vi "Main2.vi"() -> ()   [LabVIEW 2014]
uses:
  Enum State Typedef.ctl
  <vilib>/Utility/error.llb/DialogType.ctl
  <vilib>/_DAQmxBase/Internals/DAQmxBase Create Channel (AI-Voltage-Basic).vi
  <vilib>/_DAQmxBase/Internals/DAQmxBase Timing (Sample Clock).vi
  <vilib>/_DAQmxBase/Internals/DAQmxBase Read (Analog 2D DBL NChan NSamp).vi
  <vilib>/Utility/file.llb/Write To Spreadsheet File (DBL).vi
panel:
  out "State":T1
  in  "Clear Display":bool
  in  "Preview Button":bool
  out "size(s)":i32
  in  "pH":dbl
  in  "Conductivity (mS)":dbl
  out "Iterations Recorded":i32
  in  "Recording Time (seconds)":dbl
  in  "Sample Rate":i32=1000
  in  "physical channels":tag
  in  "Stop Button":bool
  out "Waveform Chart":waveform(dbl)(graph)
  in  "High Pass Filter":enum16{"500", "1k", "5k", "10k", "20k"}(ring)
  in  "Low Pass Filter":enum16{"0.1", "1.0", "10", "100", "300"}(ring)
  in  "Gain":enum16{"x100", "x1000", "x10k"}(ring)
  in  "Notch Filter":bool
  in  "Amplifier Model":u16(ring) items=["Select a Model", "AM 1700", "BMA 200"]
  in  "AC/DC Switch":bool
  in  "Temperature (deg C)":dbl
  in  "User Comments":string
  out "Start Time hr/min":string
  out "Date mm/dd/yy":string
  in  "Species":string
  in  "Exit Button":bool
  in  "Record Button":bool
  # "MSU EFISH Lab Single Channel Electronic Pulse Recorder"
  # "Must enter numbers into here before you run"
  # "Blue for On\nOrange for Off"
  # "DC"
  # "AC"
  # "Blue for AC and Orange for DC"
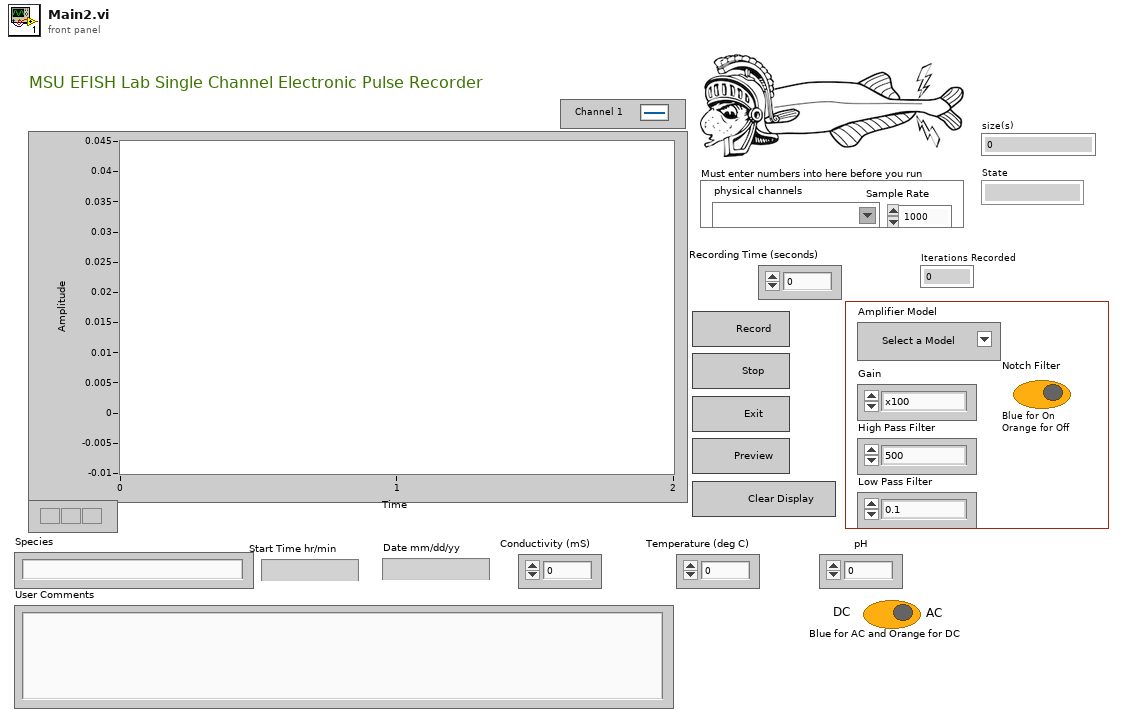
[diagram p1: front panel]
types:
  T1 = typedef "Enum State Typedef.ctl" = enum16{"", "Prepreview Handling", "Clear Display", "Preview Data", "Stop", "Exit", "Record", "Create File"}
  T2 = typedef "DialogType.ctl" = u16
  T3 = cluster{"High Pass Filter":enum16{"500", "1k", "5k", "10k", "20k"}, "Gain":enum16{"x100", "x1000", "x10k"}, "Low Pass Filter":enum16{"0.1", "1.0", "10", "100", "300"}, "Amplifier Model":u16, "Notch Filter":bool, "AC/DC Switch":bool, "Temperature (deg C)":dbl, "Conductivity (mS)":dbl, "pH":dbl, "User Comments":string, "Species":string}
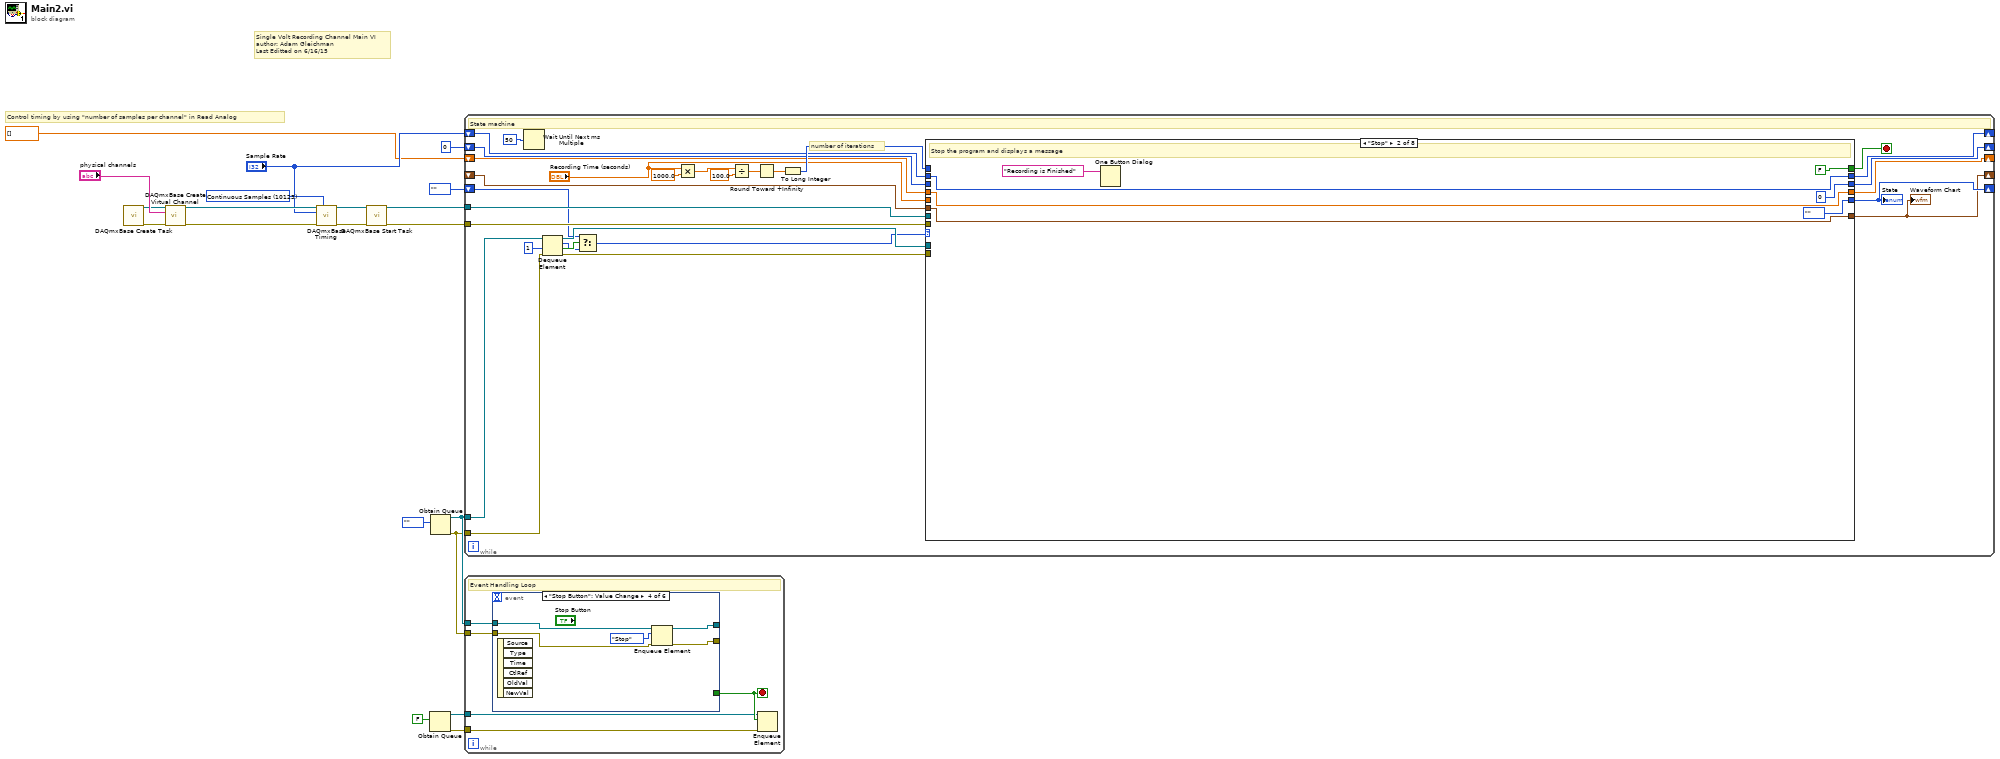
[diagram p0: block diagram]
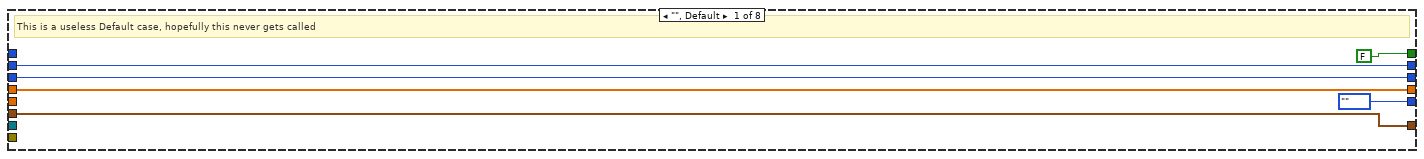
[diagram p2: hidden frame]
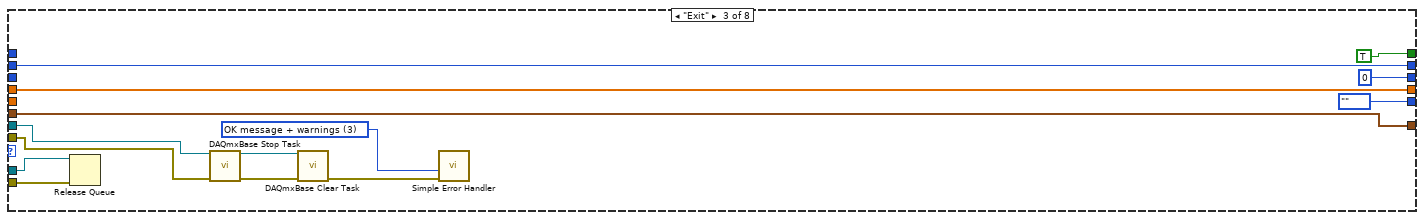
[diagram p3: hidden frame]
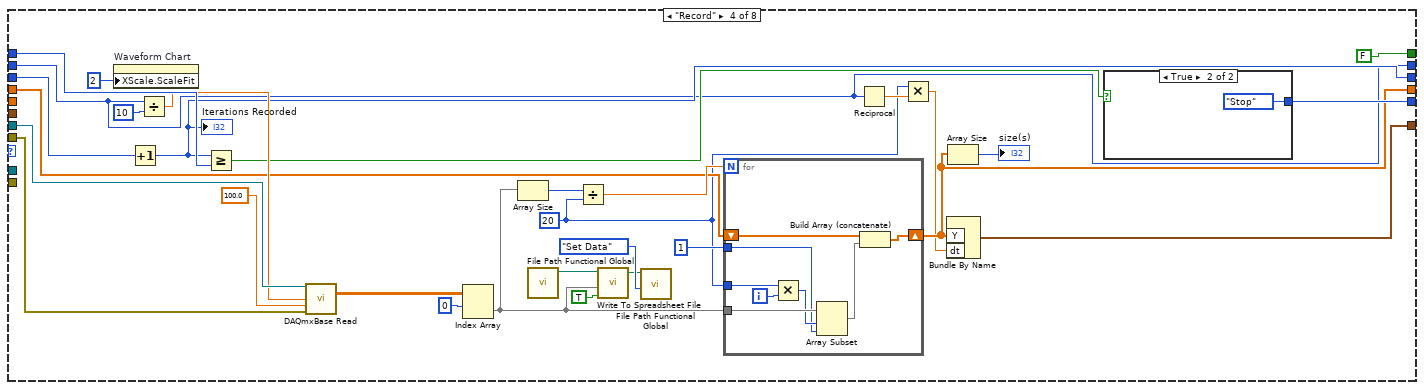
[diagram p4: hidden frame]
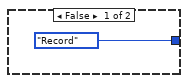
[diagram p5: hidden frame]
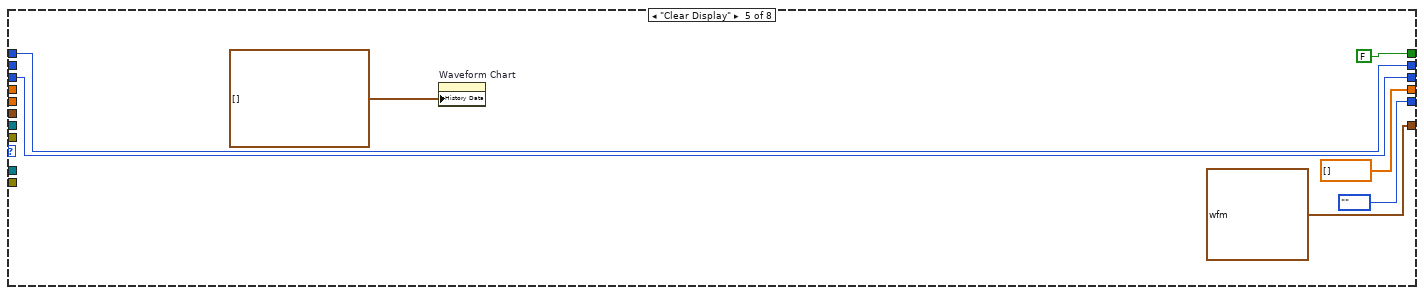
[diagram p6: hidden frame]
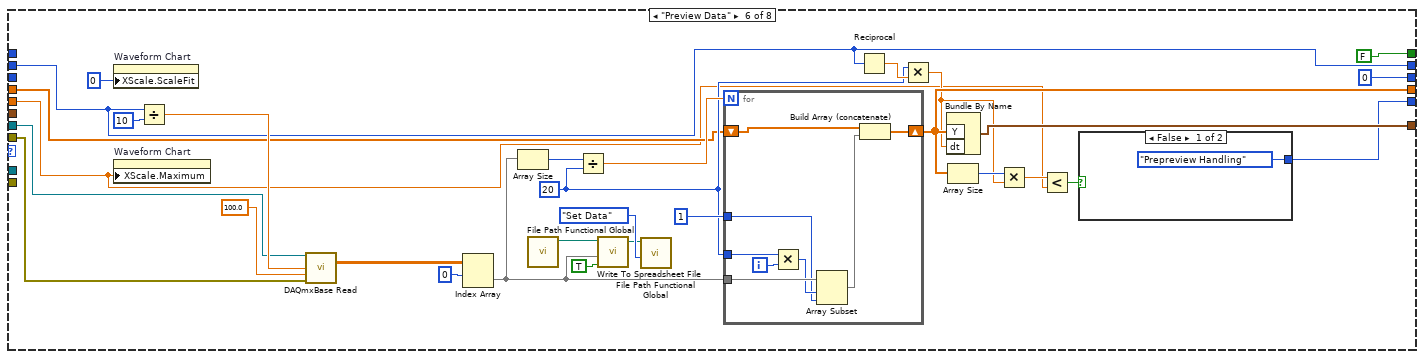
[diagram p7: hidden frame]
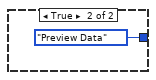
[diagram p8: hidden frame]
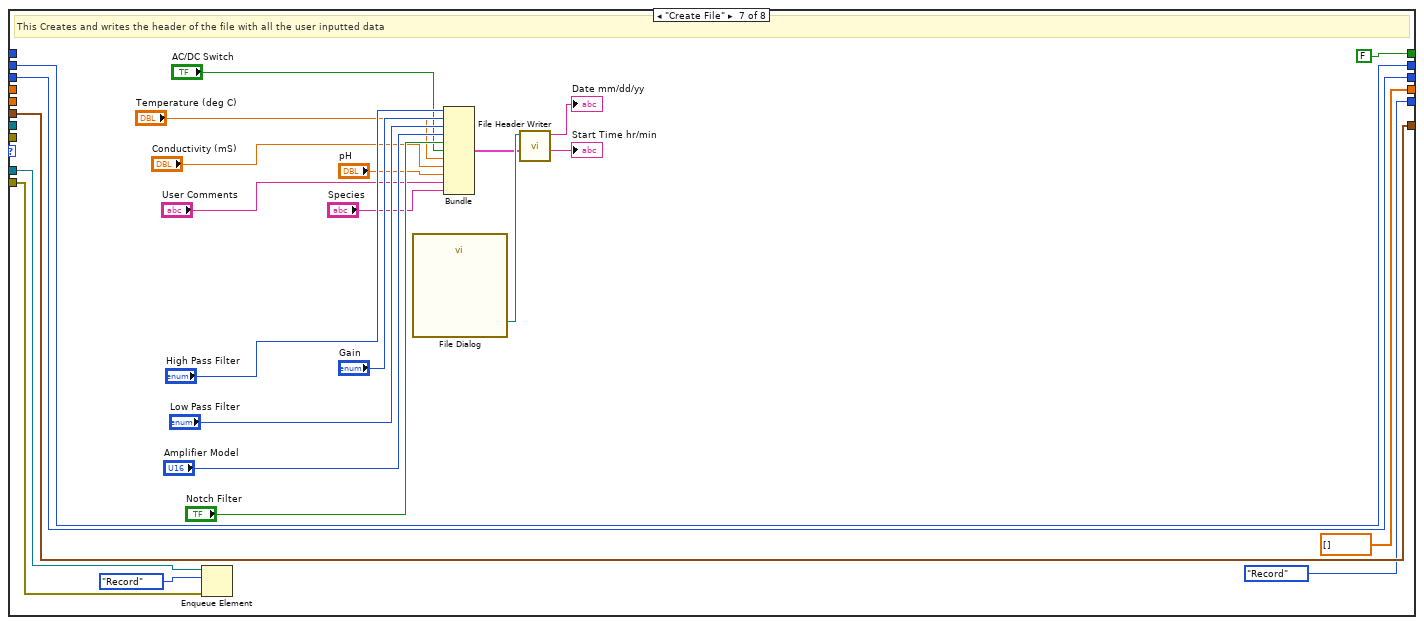
[diagram p9: hidden frame]
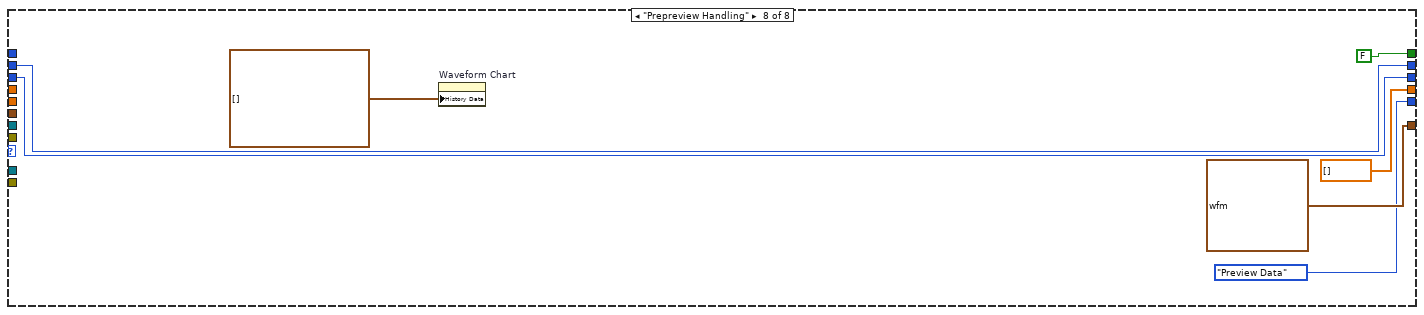
[diagram p10: hidden frame]
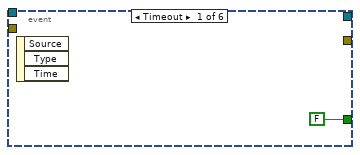
[diagram p11: hidden frame]
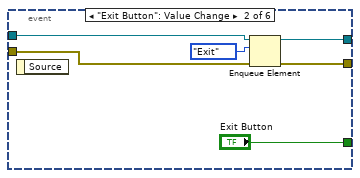
[diagram p12: hidden frame]
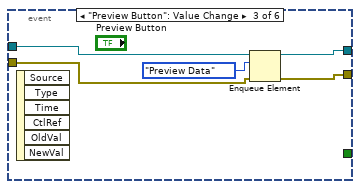
[diagram p13: hidden frame]
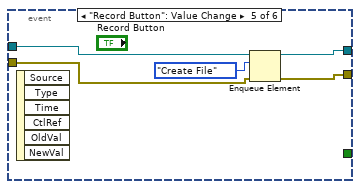
[diagram p14: hidden frame]
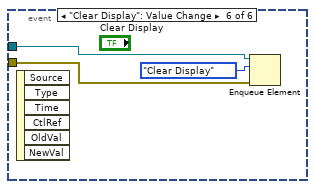
[diagram p15: hidden frame]
diagram:
  w12 = 10123 items=["Finite Samples"=10178, "Continuous Samples"=10123, "Hardware Timed Single Point"=12522] ("sample mode")
  # "Single Volt Recording Channel Main VI\nauthor: Adam Gleichman\nLast Editted on 6/16/15"
  # "Control timing by using \"number of samples per channel\" in Read Analog"
  n1 = call <vilib>:"DAQmxBase Create Task.vi"() -> ("task out"=w16:refnum<k21>, "error out"=w15:errorcluster)  [unwired: 14 in]
  n2 = call-poly <vilib>:"DAQmxBase Create Virtual Channel.vi"("task in"=w16, "physical channels"="physical channels", "error in"=w15) -> ("task out"=w14:refnum<k21>, "error out"=w13:errorcluster)  [unwired: 11 in]
  n3 = call-poly <vilib>:"DAQmxBase Timing.vi"("task/channels in"=w14, "sample mode"=w12, "rate"="Sample Rate", "error in"=w13) -> ("task out"=w11:refnum<k21>, "error out"=w10:errorcluster)  [unwired: 10 in]
  n4 = call <vilib>:"DAQmxBase Start Task.vi"("task/channels in"=w11, "error in"=w10) -> ("task out"=w8:refnum<k21>, "error out"=w9:errorcluster)  [unwired: 12 in]
  n5 = Obtain Queue(element data type=FALSE) -> (queue out=w2:refnum<queue>, error out=w1:errorcluster)  [unwired: 4 in, 1 out]
  n6 = Obtain Queue(element data type=Enum_State_Typedef."" ("State")) -> (queue out=w19:refnum<queue>, error out=w18:errorcluster)  [unwired: 4 in, 1 out]
  n7 = while {
    tunnel: w19 -> [w49]
    tunnel: w18 -> [w48]
    tunnel: w9 -> [w43]
    tunnel: w8 -> [w44]
    shift-right: [w35] -> _
    shift-left: 0 -> [w36]
    shift-right: [w30] -> _
    shift-left: Enum_State_Typedef."" ("State") -> [w32]
    shift-right: [w28] -> _
    shift-left: "Sample Rate" -> [w29]
    shift-right: [w22] -> _
    shift-left: dbl[] [] -> [w25]
    shift-right: [w24] -> _
    shift-left: _ -> [w23]
    stop <- w47 stop-if-true
    # "number of iterations"
    # "State machine"
    n8 = Wait Until Next ms Multiple(millisecond multiple=u32 50) -> ()  [unwired: 1 out]
    n9 = Dequeue Element(queue=w49, timeout in ms (-1)=1, error in (no error)=w48) -> (queue out=w46:refnum<queue>, element=w33:T1, timed out?=w34:bool, error out=w45:errorcluster)
    n10 = Select(t=w32, s=w34, f=w33) -> (s? t:f=w31:T1)
    n11 = Multiply(x="Recording Time (seconds)", y=1000.0) -> (x*y=w41:dbl)
    n12 = Divide(x=w41, y=100.0) -> (x/y=w39:dbl)
    n13 = Round Toward +Infinity(x=w39) -> (ceil(x): smallest int >= x=w38:dbl)
    n14 = To Long Integer(number=w38) -> (32bit integer=w37:i32)
    n15 = case shown="\"Stop\"" w31 {
      tunnel: [FALSE FALSE TRUE FALSE FALSE FALSE FALSE FALSE] -> w47
      tunnel: w46 -> [_ _ w69 _ _ _ w187 _]
      tunnel: w45 -> [_ _ w68 _ _ _ w186 _]
      tunnel: w44 -> [_ _ w73 w105 _ w135 _ _]
      tunnel: w43 -> [_ _ w72 w104 _ w134 _ _]
      tunnel: w29 -> [w52 w59 w65 w81 _ w130 w183 w189]
      tunnel: w37 -> [_ _ _ w97 w120 _ _ _]
      tunnel: w36 -> [w54 _ _ w98 w123 _ w184 w190]
      tunnel: [w54 0 0 w92 w123 0 w184 w190] -> w35
      tunnel: [Enum_State_Typedef."" ("State") Enum_State_Typedef."" ("State") Enum_State_Typedef."" ("State") w94 Enum_State_Typedef."" ("State") w132 Enum_State_Typedef."Record" ("State") Enum_State_Typedef."Preview Data" ("State")] -> w30
      tunnel: [w52 w59 w65 w81 w120 w130 w183 w189] -> w28
      tunnel: [w51 w57 w64 w85 dbl[] [] w131 dbl[] [] dbl[] []] -> w22
      tunnel: w25 -> [w51 w57 w64 w84 _ w136 _ _]
      tunnel: [w50 w56 w63 w83 waveform(dbl) {"t0"=timestamp(0 s since 1904-01-01), "dt"=1.0, "Y"=[]} w133 w171 waveform(dbl) {"t0"=timestamp(0 s since 1904-01-01), "dt"=1.0, "Y"=[]}] -> w24
      tunnel: w23 -> [w50 w56 w63 _ _ _ w171 _]
      tunnel: "Recording Time (seconds)" -> [_ _ _ _ _ w125 _ _]
      frame "", Default {
        # "This is a useless Default case, hopefully this never gets called"
      }
      frame "Stop" {
        # "Stop the program and displays a message"
        n16 = One Button Dialog(message="Recording is Finished") -> ()  [unwired: 1 in, 1 out]
      }
      frame "Exit" {
        w70 = T2 3 items=["no dialog", "OK message", "continue or stop message", "OK message + warnings", "continue/stop + warnings"] ("type of dialog (OK msg:1)")
        n17 = Release Queue(queue=w69, error in (no error)=w68) -> ()  [unwired: 1 in, 3 out]
        n18 = call <vilib>:"DAQmxBase Stop Task.vi"("task/channels in"=w73, "error in"=w72) -> ("task out"=w75:refnum<k21>, "error out"=w74:errorcluster)  [unwired: 12 in]
        n19 = call <vilib>:"DAQmxBase Clear Task.vi"("task in"=w75, "error in"=w74) -> ("error out"=w71:errorcluster)  [unwired: 13 in]
        n20 = call <vilib>:"Simple Error Handler.vi"("type of dialog (OK msg:1)"=w70, "error in (no error)"=w71) -> ()  [unwired: 3 in, 5 out]
      }
      frame "Record" {
        w79 = 20 ("y")
        n21 = property on="Waveform Chart" class="WFChart (strict)"("XScale.ScaleFit"=u8 2 ("X Scale.Scale Fit")) -> ()  [unwired: 2 in, 2 out]
        n22 = Increment(x=w98) -> (x+1=w92:i32)
        "Iterations Recorded" <- w92
        n23 = Divide(x=w81, y=10) -> (x/y=w95:dbl)
        n24 = Greater Or Equal?(x=w92, y=w97) -> (x >= y?=w93:bool)
        n25 = call-poly <vilib>:"DAQmxBase Read.vi"("task/channels in"=w105, "number of samples per channel"=w95, "timeout"=100.0, "error in"=w104) -> ("data"=w90:dbl[][])  [unwired: 9 in, 2 out]
        n26 = Index Array(array=w90, index (row)=0) -> (element=w82:dbl[])  [unwired: 1 in]
        n27 = Array Size(array=w82) -> (size(s)=w89:i32)
        n28 = call "File Path Functional Global.vi"() -> ("File Path Output"=w102:path)  [unwired: 11 in]
        n29 = Divide(x=w89, y=w79) -> (x/y=w88:dbl)
        n30 = call-poly <vilib>:"Write To Spreadsheet File.vi"("append to file? (new file:F)"=TRUE, "1D data"=w82, "file path (dialog if empty)"=w102) -> ("new file path (Not A Path if cancelled)"=w100:path)  [unwired: 5 in]
        n31 = call "File Path Functional Global.vi"("Enum"=enum16{"Get Data", "Set Data"}."Set Data", "File Path Control"=w100) -> ()  [unwired: 9 in, 1 out]
        n32 = for {
          N: w88 -> [_]
          shift-right: [w107] -> w85
          shift-left: w84 -> [w109]
          tunnel: w82 -> [w114]
          tunnel: w79 -> [w112]
          tunnel: 1 ("y") -> [w110]
          i -> [w113]
          n33 = Multiply(x=w112, y=w113) -> (x*y=w111:i32)
          n34 = Array Subset(array=w114, index=w111, length=w110) -> (w108:dbl[])
          n35 = Build Array (concatenate)(w109, w108) -> (w107:dbl[])
        }
        n36 = Reciprocal(x=w81) -> (1/x=w80:dbl)
        n37 = Multiply(x=w79, y=w80) -> (x*y=w78:dbl)
        n38 = Bundle By Name("Y"=w85, "dt"=w78) -> (w83:waveform(dbl))  [unwired: 1 in]
        n39 = Array Size(array=w85) -> (size(s)=→"size(s)":i32)
        n40 = case shown="True" w93 {
          tunnel: [Enum_State_Typedef."Record" ("State") Enum_State_Typedef."Stop" ("State")] -> w94
          frame False {
          }
          frame True {
          }
        }
      }
      frame "Clear Display" {
        n41 = property on="Waveform Chart" class="WFChart (strict)"("History Data"=waveform(dbl)[] []) -> ()  [unwired: 2 in, 2 out]
      }
      frame "Preview Data" {
        w137 = 20 ("y")
        n42 = property on="Waveform Chart" class="WFChart (strict)"("XScale.ScaleFit"=u8 0 ("X Scale.Scale Fit")) -> ()  [unwired: 2 in, 2 out]
        n43 = property on="Waveform Chart" class="WFChart (strict)"("XScale.Maximum"=w125) -> ()  [unwired: 2 in, 2 out]
        n44 = Divide(x=w130, y=10) -> (x/y=w145:dbl)
        n45 = call-poly <vilib>:"DAQmxBase Read.vi"("task/channels in"=w135, "number of samples per channel"=w145, "timeout"=100.0, "error in"=w134) -> ("data"=w143:dbl[][])  [unwired: 9 in, 2 out]
        n46 = Index Array(array=w143, index (row)=0) -> (element=w139:dbl[])  [unwired: 1 in]
        n47 = Array Size(array=w139) -> (size(s)=w142:i32)
        n48 = call "File Path Functional Global.vi"() -> ("File Path Output"=w150:path)  [unwired: 11 in]
        n49 = Divide(x=w142, y=w137) -> (x/y=w141:dbl)
        n50 = call-poly <vilib>:"Write To Spreadsheet File.vi"("append to file? (new file:F)"=TRUE, "1D data"=w139, "file path (dialog if empty)"=w150) -> ("new file path (Not A Path if cancelled)"=w148:path)  [unwired: 5 in]
        n51 = call "File Path Functional Global.vi"("Enum"=enum16{"Get Data", "Set Data"}."Set Data", "File Path Control"=w148) -> ()  [unwired: 9 in, 1 out]
        n52 = for {
          N: w141 -> [_]
          shift-right: [w156] -> w131
          shift-left: w136 -> [w158]
          tunnel: w139 -> [w163]
          tunnel: w137 -> [w161]
          tunnel: 1 ("y") -> [w159]
          i -> [w162]
          n53 = Multiply(x=w161, y=w162) -> (x*y=w160:i32)
          n54 = Array Subset(array=w163, index=w160, length=w159) -> (w157:dbl[])
          n55 = Build Array (concatenate)(w158, w157) -> (w156:dbl[])
        }
        n56 = Reciprocal(x=w130) -> (1/x=w138:dbl)
        n57 = Multiply(x=w137, y=w138) -> (x*y=w127:dbl)
        n58 = Bundle By Name("Y"=w131, "dt"=w127) -> (w133:waveform(dbl))  [unwired: 1 in]
        n59 = Array Size(array=w131) -> (size(s)=w128:i32)
        n60 = Multiply(x=w128, y=w127) -> (x*y=w126:dbl)
        n61 = Less?(x=w126, y=w125) -> (x < y?=w129:bool)
        n62 = case shown="False" w129 {
          tunnel: [Enum_State_Typedef."Prepreview Handling" ("State") Enum_State_Typedef."Preview Data" ("State")] -> w132
          frame False {
          }
          frame True {
          }
        }
      }
      frame "Create File" {
        # "This Creates and writes the header of the file with all the user inputted data"
        n63 = Enqueue Element(queue=w187, element=Enum_State_Typedef."Record", error in (no error)=w186) -> ()  [unwired: 1 in, 3 out]
        n64 = call "File Dialog"() -> ("selected path"=w168:path)  [unwired: 12 in, 3 out]
        n65 = Bundle("High Pass Filter"="High Pass Filter", "Gain"="Gain", "Low Pass Filter"="Low Pass Filter", "Amplifier Model"="Amplifier Model", "Notch Filter"="Notch Filter", "AC/DC Switch"="AC/DC Switch", "Temperature (deg C)"="Temperature (deg C)", "Conductivity (mS)"="Conductivity (mS)", "pH"="pH", "User Comments"="User Comments", "Species"="Species") -> (w167:T3)  [unwired: 1 in]
        n66 = call "File Header Writer.vi"("Data Cluster"=w167, "File Path"=w168) -> ("Start Time hr/min"=→"Start Time hr/min":string, "Date mm/dd/yy"=→"Date mm/dd/yy":string)  [unwired: 8 in]
      }
      frame "Prepreview Handling" {
        n67 = property on="Waveform Chart" class="WFChart (strict)"("History Data"=waveform(dbl)[] []) -> ()  [unwired: 2 in, 2 out]
      }
    }
    "Waveform Chart" <- w24
    "State" <- w30
  }
  n68 = while {
    tunnel: w19 -> [w199]
    tunnel: w18 -> [w198]
    tunnel: w2 -> [w196]
    tunnel: w1 -> [w195]
    stop <- w197 stop-if-true
    # "Event Handling Loop"
    n69 = event shown="[3] \"Stop Button\": Value Change" {
      selector: _ -> [_ _ _ _ _ _]
      dyn-events: _ -> [_ _ _ _ _ _]
      timeout: _ -> [_ _ _ _ _ _]
      tunnel: [FALSE ("Exit Button") "Exit Button" _ _ _ _] -> w197
      tunnel: w199 -> [_ w205 w211 w216 w221 w224]
      tunnel: w198 -> [_ w204 w210 w215 w220 w223]
      tunnel: [_ w203 w208 w213 w218 _] -> _
      tunnel: [_ w202 w207 w214 w219 _] -> _
      event Timeout {
        n70 = event-data() -> ()  [unwired: 1 in, 3 out]
      }
      event "Exit Button": Value Change {
        n71 = event-data() -> ()  [unwired: 1 in, 1 out]
        n72 = Enqueue Element(queue=w205, element=Enum_State_Typedef."Exit", error in (no error)=w204) -> (queue out=w203:refnum<queue>, error out=w202:errorcluster)  [unwired: 1 in, 1 out]
      }
      event "Preview Button": Value Change {
        n73 = event-data() -> ()  [unwired: 1 in, 6 out]
        n74 = Enqueue Element(queue=w211, element=Enum_State_Typedef."Preview Data", error in (no error)=w210) -> (queue out=w208:refnum<queue>, error out=w207:errorcluster)  [unwired: 1 in, 1 out]
      }
      event "Stop Button": Value Change {
        n75 = event-data() -> ()  [unwired: 1 in, 6 out]
        n76 = Enqueue Element(queue=w216, element=Enum_State_Typedef."Stop", error in (no error)=w215) -> (queue out=w213:refnum<queue>, error out=w214:errorcluster)  [unwired: 1 in, 1 out]
      }
      event "Record Button": Value Change {
        n77 = event-data() -> ()  [unwired: 1 in, 6 out]
        n78 = Enqueue Element(queue=w221, element=Enum_State_Typedef."Create File", error in (no error)=w220) -> (queue out=w218:refnum<queue>, error out=w219:errorcluster)  [unwired: 1 in, 1 out]
      }
      event "Clear Display": Value Change {
        n79 = event-data() -> ()  [unwired: 1 in, 6 out]
        n80 = Enqueue Element(queue=w224, element=Enum_State_Typedef."Clear Display", error in (no error)=w223) -> ()  [unwired: 1 in, 3 out]
      }
    }
    n81 = Enqueue Element(queue=w196, element=w197, error in (no error)=w195) -> ()  [unwired: 1 in, 3 out]
  }
